vi "calculate group change.vi"(8 "error in":errorcluster, 10 "Current group":string, 11 "Set group":string) -> (0 "error out":errorcluster, 1 "keystroke":string, 2 "Action":string, 3 "num changes":i32)   [LabVIEW 2018]
uses:
  CAEN globals.vi
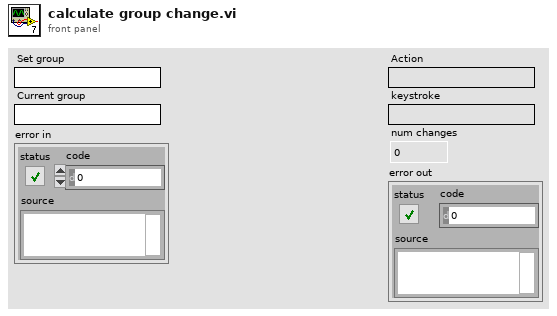
[diagram p1: front panel]
types:
  T1 = typedef "channel.ctl" = cluster{" Card.Channel":dbl, "Crate":i32}
  T2 = cluster{"Group Name":string, "Channels in Group":T1[]}[]
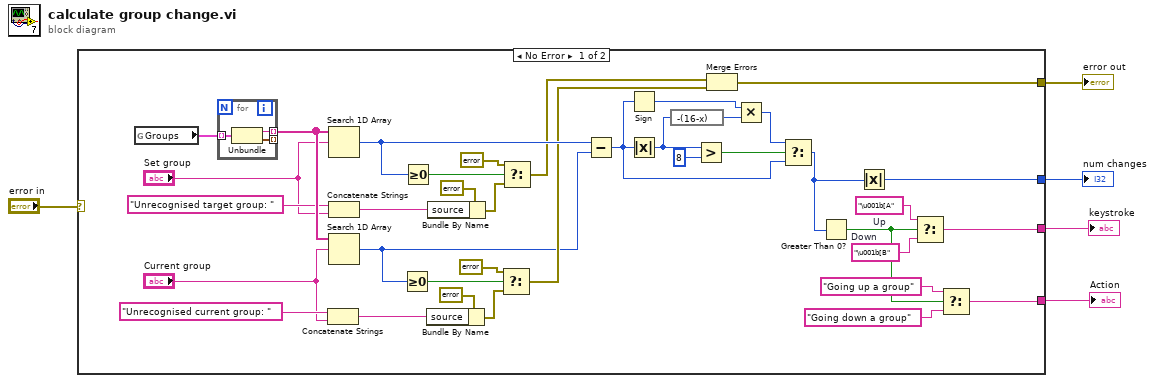
[diagram p0: block diagram]
diagram:
  n1 = case shown="No Error" "error in" {
    selector: "error in" -> [_ w46]
    tunnel: [w36 w46] -> w5
    tunnel: [w13 _] -> w3
    tunnel: [w12 _] -> w2
    tunnel: [w11 _] -> w1
    frame No Error {
      w40 = "\u001b[A"  # Up
      w41 = "\u001b[B"  # Down
      n2 = global read "CAEN globals.vi" "Groups"() -> (w14:T2)
      n3 = for {
        tunnel: w14 -> [w45] mode=indexing
        tunnel: [w44] -> w42 mode=indexing
        tunnel: [w43] -> _ mode=indexing
        n4 = Unbundle(w45) -> ("Group Name"=w44:string, "Channels in Group"=w43:T1[])
      }
      n5 = Concatenate Strings("Unrecognised current group: " ("Up"), "Current group") -> (w30:string)
      n6 = Search 1D Array(1D array=w42, element="Set group") -> (index of element=w19:i32)  [unwired: 1 in]
      n7 = Concatenate Strings("Unrecognised target group: " ("Up"), "Set group") -> (w25:string)
      n8 = Search 1D Array(1D array=w42, element="Current group") -> (index of element=w16:i32)  [unwired: 1 in]
      n9 = Greater Or Equal To 0?(x=w16) -> (x >= 0?=w33:bool)
      n10 = Greater Or Equal To 0?(x=w19) -> (x >= 0?=w22:bool)
      n11 = Bundle By Name(cluster=errorcluster {"status"=TRUE, "code"=0, "source"="Unrecognised current group"} ("t"), "source"=w30) -> (w27:errorcluster)
      n12 = Bundle By Name(cluster=errorcluster {"status"=TRUE, "code"=0, "source"="Unrecognised current group"} ("t"), "source"=w25) -> (w26:errorcluster)
      n13 = Select(t=errorcluster {"status"=FALSE, "code"=0, "source"=""}, s=w33, f=w27) -> (s? t:f=w17:errorcluster)
      n14 = Select(t=errorcluster {"status"=FALSE, "code"=0, "source"=""}, s=w22, f=w26) -> (s? t:f=w18:errorcluster)
      n15 = Subtract(x=w19, y=w16) -> (x-y=w6:i32)
      n16 = Sign(1:w6) -> (0:w7:i32)
      n17 = Absolute Value(x=w6) -> (abs(x)=w10:i32)
      n18 = expression code="-(16-x)"(w10) -> (w9:i32)
      n19 = Greater?(x=w10, y=8) -> (0:w35:bool)
      n20 = Merge Errors(w18, w17) -> (w36:errorcluster)
      n21 = Multiply(x=w7, y=w9) -> (x*y=w8:i32)
      n22 = Select(t=w8, s=w35, f=w6) -> (s? t:f=w15:i32)
      n23 = Greater Than 0?(x=w15) -> (x > 0?=w38:bool)
      n24 = Absolute Value(x=w15) -> (abs(x)=w13:i32)
      n25 = Select(t=w40, s=w38, f=w41) -> (s? t:f=w12:string)
      n26 = Select(t="Going up a group" ("Up"), s=w38, f="Going down a group" ("Up")) -> (s? t:f=w11:string)
    }
    frame Error {
    }
  }
  "error out" <- w5
  "num changes" <- w3
  "keystroke" <- w2
  "Action" <- w1
